vi "getVariaStatusBits.vi"(8 "error in (no error)":errorcluster, 11 "COMport":string="COM6") -> (0 "error out":errorcluster, 1 "statusBitCluster":T1, 2 "bitMaskDecimal":i32)   [LabVIEW 2015]
panel:
  out "Status Bitmask":u16 format="%b"
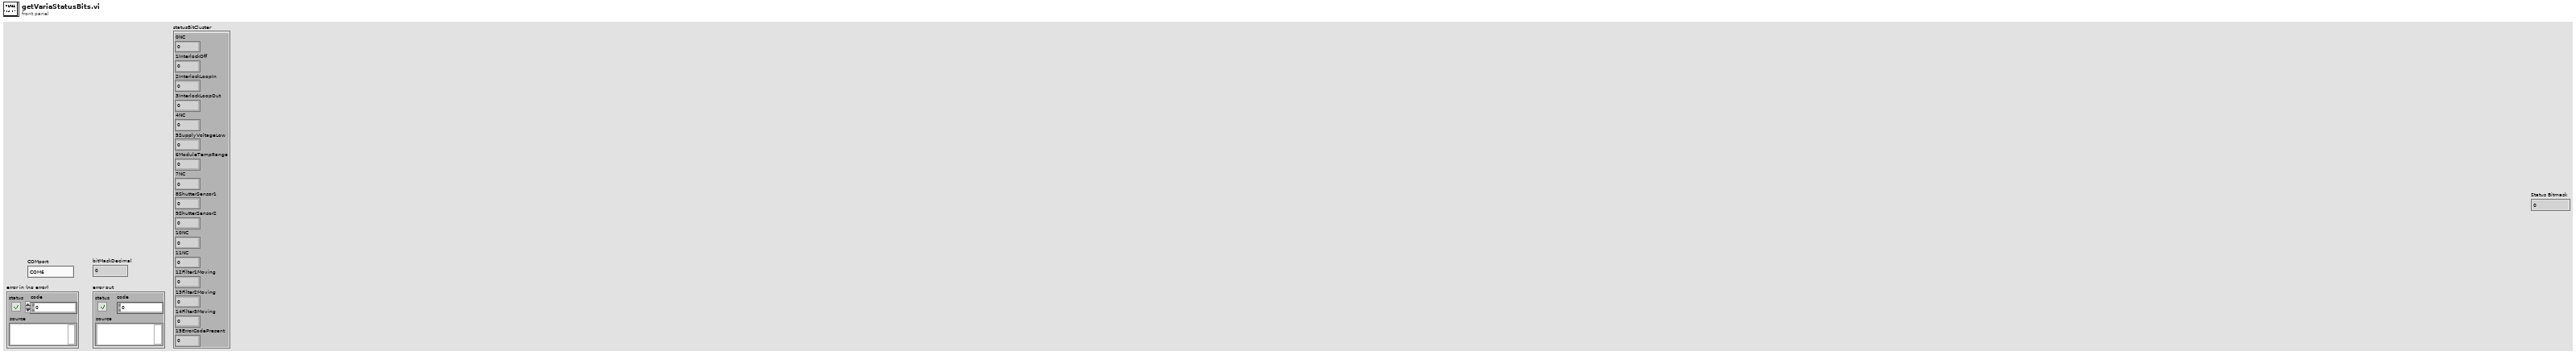
[diagram p1: front panel]
types:
  T1 = cluster{"0NC":i16, "1InterlockOff":i16, "2InterlockLoopIn":i16, "3InterlockLoopOut":i16, "4NC":i16, "5SupplyVoltageLow":i16, "6ModuleTempRange":i16, "7NC":i16, "8ShutterSensor1":i16, "9ShutterSensor2":i16, "10NC":i16, "11NC":i16, "12Filter1Moving":i16, "13Filter2Moving":i16, "14Filter3Moving":i16, "15ErrorCodePresent":i16}
  T2 = cluster{"[0]":i16, "[1]":i16, "[2]":i16, "[3]":i16, "[4]":i16, "[5]":i16, "[6]":i16, "[7]":i16, "[8]":i16, "[9]":i16, "[10]":i16, "[11]":i16, "[12]":i16, "[13]":i16, "[14]":i16, "[15]":i16}
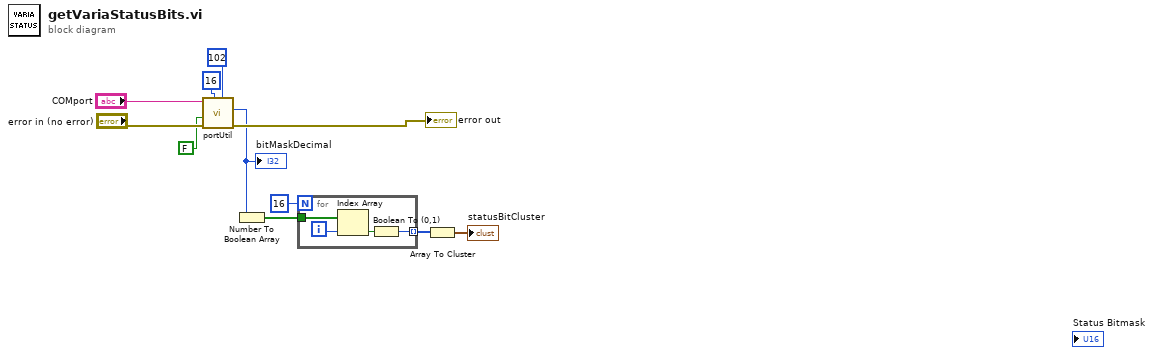
[diagram p0: block diagram]
diagram:
  n1 = call "portUtil.vi"("Register"=u8 102, "Destination"=u8 16, "error in (no error)"="error in (no error)", "WriteNotRead"=FALSE, "COMport"="COMport") -> ("error out"=→"error out":errorcluster, "Long"=w3:i32)  [unwired: 4 in, 1 out]
  "bitMaskDecimal" <- w3
  n2 = Number To Boolean Array(number=w3) -> (Boolean array=w6:bool[])
  n3 = for {
    N: 16 -> [_]
    tunnel: w6 -> [w15]
    tunnel: [w12] -> w4 mode=indexing
    i -> [w14]
    n4 = Index Array(array=w15, index=w14) -> (element=w13:bool)
    n5 = Boolean To (0,1)(Boolean=w13) -> (0, 1=w12:i16)
  }
  n6 = Array To Cluster(array=w4) -> (cluster=→"statusBitCluster":T2)
